vi "Get Job Attributes Numeric.vi"(10 "Attribute":string, 11 "JOB Attributes":string[][](array[string])) -> (3 "Cell String":u16)   [LabVIEW 2021]
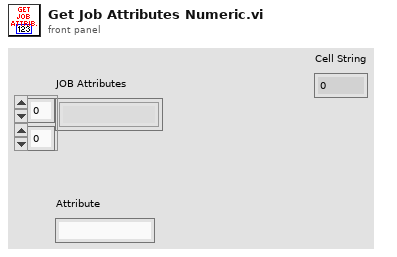
[diagram p1: front panel]
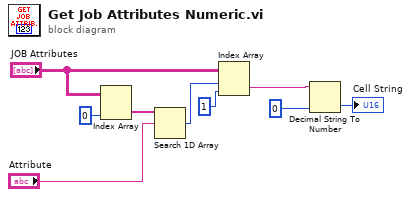
[diagram p0: block diagram]
diagram:
  n1 = Index Array(array="JOB Attributes", index (col)=0 ("disabled index (col)")) -> (element=w5:string[])  [unwired: 1 in]
  n2 = Search 1D Array(1D array=w5, element="Attribute") -> (index of element=w8:i32)  [unwired: 1 in]
  n3 = Index Array(array="JOB Attributes", index (row)=w8, index (col)=1 ("disabled index (col)")) -> (element=w2:string)
  n4 = Decimal String To Number(string=w2, default (0L)=u16 0 ("default (0 I32)")) -> (number=→"Cell String":u16)  [unwired: 1 in, 1 out]
